vi "CirculationCtl.vi"(0 "Pump":bool, 1 "OnTime [min]":u8, 3 "P-4 Drehzahl [%]":u8, 4 "OffTime [min]":u8, 5 "error in":errorcluster, 6 "enable":bool, 7 "shiftReg[ms]":u64, 9 "Actual Start [ms]":i64, 10 "Zirkulationgeschw.  [l/min]":dbl, 11 "DFS-1 [l/min]":dbl, 12 "Valve":bool) -> (13 "error out":errorcluster, 14 "Pump":bool, 15 "Valve":bool, 18 "P-4 Drehzahl [%]":dbl, 19 "shiftReg[ms]":u64)   [LabVIEW 2011]
uses:
  <vilib>/functionblocks/Control/PID/PID.vi
  <vilib>/functionblocks/FB Property/FB Overlay DBL.ctl
  <vilib>/functionblocks/FB Core/FB Core.xnode
  <vilib>/functionblocks/NI_FunctionBlock Libraries.lvlib
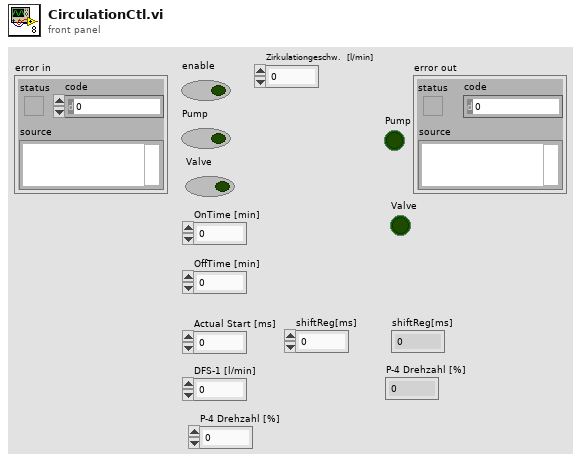
[diagram p1: front panel]
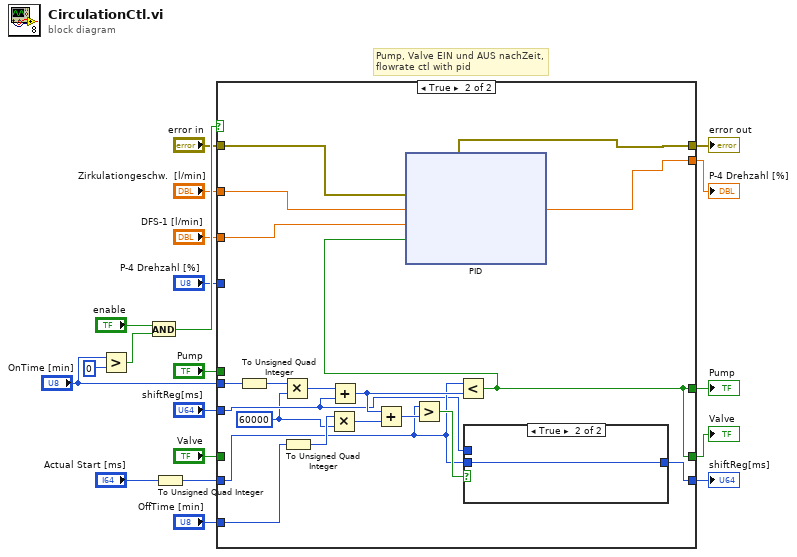
[diagram p0: block diagram]
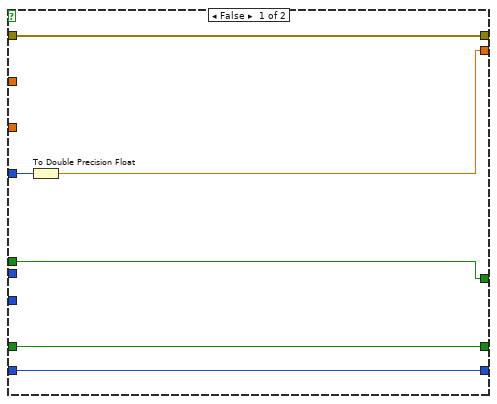
[diagram p2: hidden frame]
diagram:
  # "Pump, Valve EIN und AUS nachZeit,\nflowrate ctl with pid"
  n1 = Greater?(x="OnTime [min]", y=u8 0) -> (0:w19:bool)
  n2 = And(x="enable", y=w19) -> (x .and. y?=w18:bool)
  n3 = To Unsigned Quad Integer(1:"Actual Start [ms]") -> (0:w9:u64)
  n4 = case shown="True" w18 {
    tunnel: w9 -> [w26 w36]
    tunnel: "OnTime [min]" -> [_ w43]
    tunnel: "OffTime [min]" -> [_ w41]
    tunnel: [w25 w30] -> w14
    tunnel: "shiftReg[ms]" -> [_ w34]
    tunnel: [w26 w35] -> w12
    tunnel: "Pump" -> [w25 _]
    tunnel: [w24 w30] -> w8
    tunnel: "Valve" -> [w24 _]
    tunnel: "P-4 Drehzahl [%]" -> [w23 _]
    tunnel: "DFS-1 [l/min]" -> [_ w28]
    tunnel: [w22 w27] -> w4
    tunnel: "Zirkulationgeschw.  [l/min]" -> [_ w29]
    tunnel: "error in" -> [w21 w31]
    tunnel: [w21 w32] -> w1
    frame False {
      n5 = To Double Precision Float(number=w23) -> (double precision float=w22:dbl)
    }
    frame True {
      w33 = u64 60000 ("y")
      n6 = To Unsigned Quad Integer(1:w43) -> (0:w44:u64)
      n7 = Multiply(x=w44, y=w33) -> (x*y=w45:u64)
      n8 = To Unsigned Quad Integer(1:w41) -> (0:w42:u64)
      n9 = Multiply(x=w42, y=w33) -> (x*y=w40:u64)
      n10 = Add(x=w45, y=w34) -> (x+y=w39:u64)
      n11 = Add(x=w39, y=w40) -> (x+y=w38:u64)
      n12 = Greater?(x=w36, y=w38) -> (0:w37:bool)
      n13 = Less?(x=w36, y=w39) -> (x < y?=w30:bool)
      n14 = xnode "PID"("error in"=w31, "setpoint"=w29, "process variable"=w28, "auto? (T)"=w30) -> ("error out"=w32:errorcluster, "output"=w27:dbl)  [unwired: 1 in]
      n15 = case shown="True" w37 {
        tunnel: w36 -> [_ w113]
        tunnel: [w112 w113] -> w35
        tunnel: w34 -> [w112 _]
        frame False {
        }
        frame True {
        }
      }
    }
  }
  "Pump" <- w14
  "shiftReg[ms]" <- w12
  "Valve" <- w8
  "P-4 Drehzahl [%]" <- w4
  "error out" <- w1
